vi "IMF_determination.vi"(1 "h(t)":dbl[](array[numeric]), 2 "original signal":dbl[](array[numeric])) -> (0 "x .and. y?":bool)   [LabVIEW 2018]
panel:
  out "Numeric 3":dbl
  out "Numeric 2":dbl
  out "Numeric":dbl
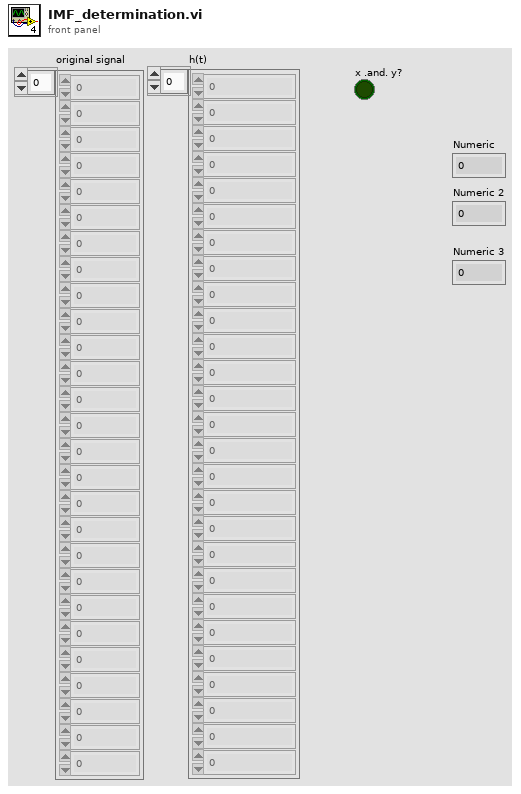
[diagram p1: front panel]
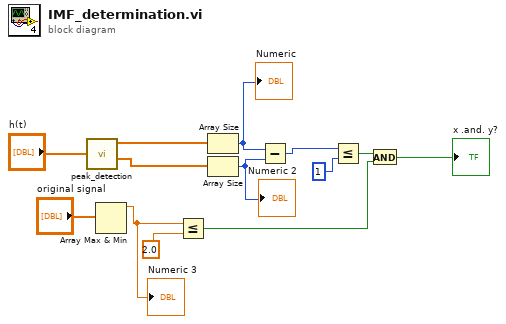
[diagram p0: block diagram]
diagram:
  n1 = call "peak_detection.vi"("Array"="h(t)") -> ("upper"=w8:dbl[], "lower"=w7:dbl[])  [unwired: 2 out]
  n2 = Array Max & Min(array="original signal") -> (max value=w1:dbl)  [unwired: 3 out]
  "Numeric 3" <- w1
  n3 = Less Or Equal?(x=w1, y=2.0) -> (x <= y?=w4:bool)
  n4 = Array Size(array=w8) -> (size(s)=w2:i32)
  "Numeric" <- w2
  n5 = Array Size(array=w7) -> (size(s)=w3:i32)
  "Numeric 2" <- w3
  n6 = Subtract(x=w2, y=w3) -> (x-y=w13:i32)
  n7 = Less Or Equal?(x=w13, y=1) -> (x <= y?=w11:bool)
  n8 = And(x=w11, y=w4) -> (x .and. y?=→"x .and. y?":bool)
